vi "stars.vi"(1 "n":i32) -> (0 "n stars":string)   [LabVIEW 2010, in "password.xctl"]
uses:
  password.xctl
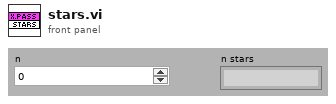
[diagram p1: front panel]
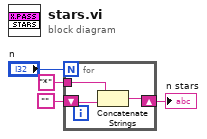
[diagram p0: block diagram]
diagram:
  n1 = for {
    N: "n" -> [_]
    shift-right: [w5] -> w4
    shift-left: "" -> [w7]
    tunnel: "*" -> [w6]
    n2 = Concatenate Strings(w6, w7) -> (w5:string)
  }
  "n stars" <- w4
